vi "Add Sensor to Tree.vi"(4 "Channel#":u16, 5 "Connected?":bool, 6 "\"Add Item\" Tag":string, 7 "Instrument Group Tag (Parent)":string, 8 "error in (no error)":errorcluster, 9 "VISA Res":refnum<visa-resource-name>, 10 "Name":string, 11 "TreeControl in":refnum<vi>) -> (0 "error out":errorcluster, 3 "Tree out":refnum<vi>)   [LabVIEW 2018]
uses:
  TypeDefs/Tree Item Type.ctl
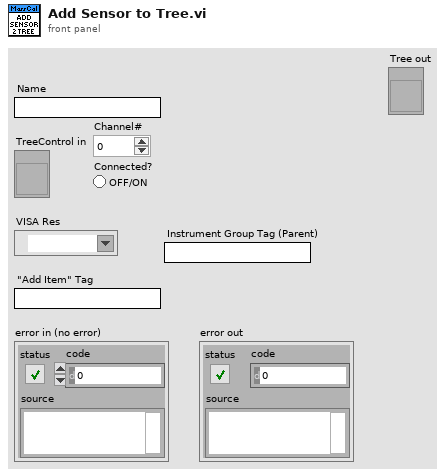
[diagram p1: front panel]
types:
  T1 = typedef "Test Manager Tree Tag.ctl" = cluster{"ItemType":T2, "VISA Resource":refnum<visa-resource-name>, "Name":string, "Channel #":u16, "ComparatorID":u16}
  T2 = typedef "Tree Item Type.ctl" = enum16{"Comparator", "Temp Group", "Press Group", "Hygro Group", "Thermometer", "PressureTransducer", "Hygrometers", "Add Comparator", "Add Thermometer", "Add Barometer", "Add Hygrometer"}
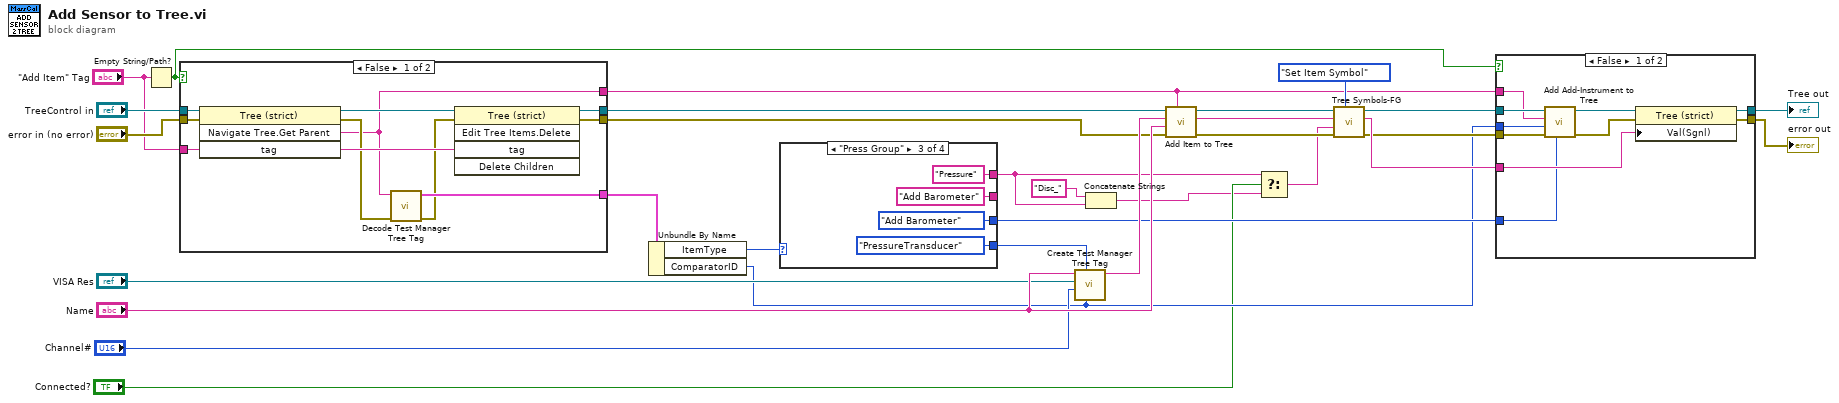
[diagram p0: block diagram]
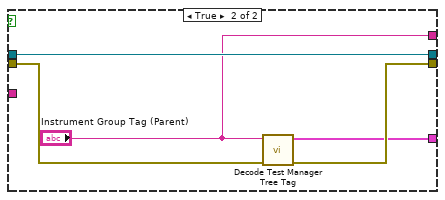
[diagram p3: hidden frame]
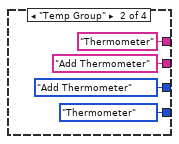
[diagram p5: hidden frame]
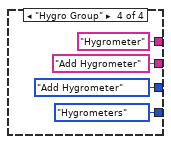
[diagram p6: hidden frame]
diagram:
  n1 = Empty String/Path?(string/path="\"Add Item\" Tag") -> (empty?=w6:bool)
  n2 = case shown="False" w6 {
    tunnel: [w40 w43] -> w25
    tunnel: "error in (no error)" -> [w39 w45]
    tunnel: [w38 w41] -> w18
    tunnel: "TreeControl in" -> [w37 w43]
    tunnel: "\"Add Item\" Tag" -> [w35 _]
    tunnel: [w32 "Instrument Group Tag (Parent)"] -> w8
    tunnel: [w31 w44] -> w13
    frame False {
      n3 = invoke class="Tree (strict)" method="Navigate Tree.Get Parent"(reference=w37, error in=w39, "tag"=w35) -> (reference out=w36:refnum<vi>, error out=w34:errorcluster, "Navigate Tree:Get Parent"=w32:string)  [unwired: 1 in, 1 out]
      n4 = call "Decode Test Manager Tree Tag.vi"("error in (no error)"=w34, "Tag"=w32) -> ("error out"=w33:errorcluster, "Test Manager Tree Tag"=w38:T1)  [unwired: 8 in]
      n5 = invoke class="Tree (strict)" method="Edit Tree Items.Delete"(reference=w36, error in=w33, "tag"=w35) -> (reference out=w40:refnum<vi>, error out=w31:errorcluster)  [unwired: 2 in, 3 out]
    }
    frame True {
      n6 = call "Decode Test Manager Tree Tag.vi"("error in (no error)"=w45, "Tag"="Instrument Group Tag (Parent)") -> ("error out"=w44:errorcluster, "Test Manager Tree Tag"=w41:T1)  [unwired: 8 in]
    }
  }
  n7 = Unbundle By Name(w18) -> ("ItemType"=w15:T2, "ComparatorID"=w7:u16)
  n8 = case shown="\"Press Group\"" w15 {
    tunnel: [_ "Thermometer" ("Symbol Name") "Pressure" ("Symbol Name") "Hygrometer" ("Symbol Name")] -> w2
    tunnel: [_ "Add Thermometer" ("Item Name") "Add Barometer" ("Item Name") "Add Hygrometer" ("Item Name")] -> _
    tunnel: [_ Tree_Item_Type."Add Thermometer" ("ItemType") Tree_Item_Type."Add Barometer" ("ItemType") Tree_Item_Type."Add Hygrometer" ("ItemType")] -> w9
    tunnel: [_ Tree_Item_Type."Thermometer" ("ItemType") Tree_Item_Type."PressureTransducer" ("ItemType") Tree_Item_Type."Hygrometers" ("ItemType")] -> w14
    frame "Comparator", Default {
    }
    frame "Temp Group" {
    }
    frame "Press Group" {
    }
    frame "Hygro Group" {
    }
  }
  n9 = call "Create Test Manager Tree Tag.vi"("Comparator ID"=w7, "ItemType"=w14, "Channel #"="Channel#", "VISA Resource"="VISA Res", "Name"="Name") -> ("Tag"=w26:string)  [unwired: 4 in, 2 out]
  n10 = Concatenate Strings("Disc_" ("string"), w2) -> (w3:string)
  n11 = call "Add Item to Tree.vi"("Parent Tag"=w8, "error in (no error)"=w13, "Item Name"="Name", "Item Tag"=w26, "Tree Ref"=w25) -> ("error out"=w28:errorcluster, "Item Tag out"=w29:string, "reference out"=w27:refnum<vi>)  [unwired: 3 in, 1 out]
  n12 = Select(t=w2, s="Connected?", f=w3) -> (s? t:f=w1:string)
  n13 = call "Tree Symbols-FG.vi"("Actions"=enum16{"Init Symbols", "Set Item Symbol"}."Set Item Symbol", "error in (no error)"=w28, "Symbol Name"=w1, "Item Tag"=w29, "Tree Ref"=w27) -> ("error out"=w11:errorcluster, "Item Tag out"=w22:string, "Tree Ref out"=w10:refnum<vi>)  [unwired: 4 in]
  n14 = case shown="False" w6 {
    tunnel: w22 -> [w67 _]
    tunnel: [w66 w68] -> w21
    tunnel: [w65 w69] -> w20
    tunnel: w11 -> [w64 w68]
    tunnel: w10 -> [w62 w69]
    tunnel: w9 -> [w60 _]
    tunnel: w8 -> [w59 _]
    tunnel: w7 -> [w58 _]
    frame False {
      n15 = call "Add Add-Instrument to Tree.vi"("ItemType"=w60, "error in (no error)"=w64, "#ofComparators (New ComparatorID)"=w58, "Instrument Group Tag in"=w59, "TreeControl in"=w62) -> ("error out"=w63:errorcluster, "TreeControl out"=w61:refnum<vi>)  [unwired: 4 in, 1 out]
      n16 = property class="Tree (strict)"(reference=w61, error in=w63, "Val(Sgnl)"=w67) -> (reference out=w65:refnum<vi>, error out=w66:errorcluster)
    }
    frame True {
    }
  }
  "error out" <- w21
  "Tree out" <- w20
